vi "CTRE_Phoenix_MotorControl_StartMotionProfile.vi"(7 "BufferedTrajectoryPointStream_DevRef":T2, 8 "error in":errorcluster, 9 "Control Mode":T1=6 items=["MotionProfile"=6, "MotionProfileArc"=10], 10 "minBufferedPts":u32, 11 "PhoenixMotorControlDevRef":T3={"DeviceStatus"={"status"=FALSE, "code"=0, "source"=""}, "Type"=enum."PWM", "PWM"={"PWM Channel"=enum."Invalid", "DeadBand"={"Name"="", "maxPositivePwm"=0, "minPositivePwm"=0, "centerPwm"=0, "maxNegativePwm"=0, "minNegativePwm"=0, "angularRange"=0}}, "CAN"={"Device Number"=0, "SetOutput VI Ref"=variant(enum8{"Percent VBus", "Current", "Speed", "Position", "Voltage"} enum."Percent VBus"), "GetOutput VI Ref"=variant(refnum<k1> refnum), "Enable VI Ref"=variant(dbl 12.0), "Disable VI Ref"=variant(enum8{"Percent VBus", "Speed", "Position", "Slave", "Unchanged / Invalid", "Voltage Compensation", "Current", "Motion Profile"} enum."Percent VBus"), "Data"=variant}, "Invert"=FALSE, "DIO PWM"={"PWM \"Enable\" Channel"=enum."Invalid", "DIOChannel"=enum."Invalid", "PWM Rate"=0.0}}) -> (0 "error out":errorcluster, 3 "PhoenixMotorControlDevRef":T3={"DeviceStatus"={"status"=FALSE, "code"=0, "source"=""}, "Type"=enum."PWM", "PWM"={"PWM Channel"=enum."Invalid", "DeadBand"={"Name"="", "maxPositivePwm"=0, "minPositivePwm"=0, "centerPwm"=0, "maxNegativePwm"=0, "minNegativePwm"=0, "angularRange"=0}}, "CAN"={"Device Number"=0, "SetOutput VI Ref"=variant(enum8{"Percent VBus", "Current", "Speed", "Position", "Voltage"} enum."Percent VBus"), "GetOutput VI Ref"=variant(refnum<k1> refnum), "Enable VI Ref"=variant(dbl 12.0), "Disable VI Ref"=variant(enum8{"Percent VBus", "Speed", "Position", "Slave", "Unchanged / Invalid", "Voltage Compensation", "Current", "Motion Profile"} enum."Percent VBus"), "Data"=variant}, "Invert"=FALSE, "DIO PWM"={"PWM \"Enable\" Channel"=enum."Invalid", "DIOChannel"=enum."Invalid", "PWM Rate"=0.0}})   [LabVIEW 2018]
doc: "Simple one-shot firing of a complete MP.\nStarting in 2019, MPs can be fired by building a Buffered Trajectory Point Stream, and calling this routine.\n\nOnce called, the motor controller software will automatically ...\n[1] Clear the firmware buffer of trajectory points.\n[2] Clear the underrun flags\n[3] Reset an index within the Buffered Trajectory Point Stream (so that the same profile can be run again and again).\n[4] Start a background thread to manage MP streaming (if not already running).\n[5a] If current control mode already matches motionProfControlMode, set MPE Output to \"Hold\".\n[5b] If current control mode does not matches motionProfControlMode, apply motionProfControlMode and set MPE Output to \"Disable\".\n[6] Stream the trajectory points into the device's firmware buffer.\n[7] Once motor controller has at least minBufferedPts worth in the firmware buffer, MP will automatically start (MPE Output set to \"Enable\").\n[8] Wait until MP finishes, then transitions the Motion Profile Executor's output to \"Hold\".\n[9] IsMotionProfileFinished() will now return true.\n\nCalling application can use IsMotionProfileFinished() to determine when internal state machine reaches [7].\nCalling application can cancel MP by calling set(). Otherwise do not call set() until MP has completed.\n\nThe legacy API from previous years requires the calling application to pass points via the ProcessMotionProfileBuffer and PushMotionProfileTrajectory.\nThis is no longer required if using this StartMotionProfile/IsMotionProfileFinished API.\n\n <b>Buffered Trajectory Point Stream</b> A buffer that will be used to stream the trajectory points. Caller can fill this container with the entire trajectory point, regardless of size.\n <b>minBufferedPts</b> Minimum number of firmware buffered points before starting MP. \n Do not exceed device's firmware buffer capacity or MP will never fire (120 for Motion Profile, or 60 for Motion Profile Arc).\n Recommendation value for this would be five to ten samples depending on timeDur of the trajectory point.\n <b>motionProfControlMode</b> Pass MotionProfile or MotionProfileArc."
uses:
  <vilib>/Rock Robotics/WPI/MotorControl/WPI_MotorControlDeviceRef.ctl
  <vilib>/Rock Robotics/WPI/MotorControl/WPI_MotorControlType.ctl
  <vilib>/Rock Robotics/SystemInterfaces/DIO/FPGA_DIOPWMChannel.ctl
  <vilib>/Rock Robotics/WPI/PWM/WPI_PWMDeadband.ctl
  <vilib>/Rock Robotics/SystemInterfaces/DIO/FPGA_DIOChannel.ctl
  <vilib>/Rock Robotics/WPI/ThirdParty/Phoenix-LabVIEW/Motor Controller/Controls/CTRE_Phoenix_MotorControl_BufferedTrajectoryPointStream_DeviceRef.ctl
  <vilib>/Rock Robotics/WPI/ThirdParty/Phoenix-LabVIEW/Motor Controller/Controls/CTRE_Phoenix_MotorControl_MotionProfileControlMode.ctl
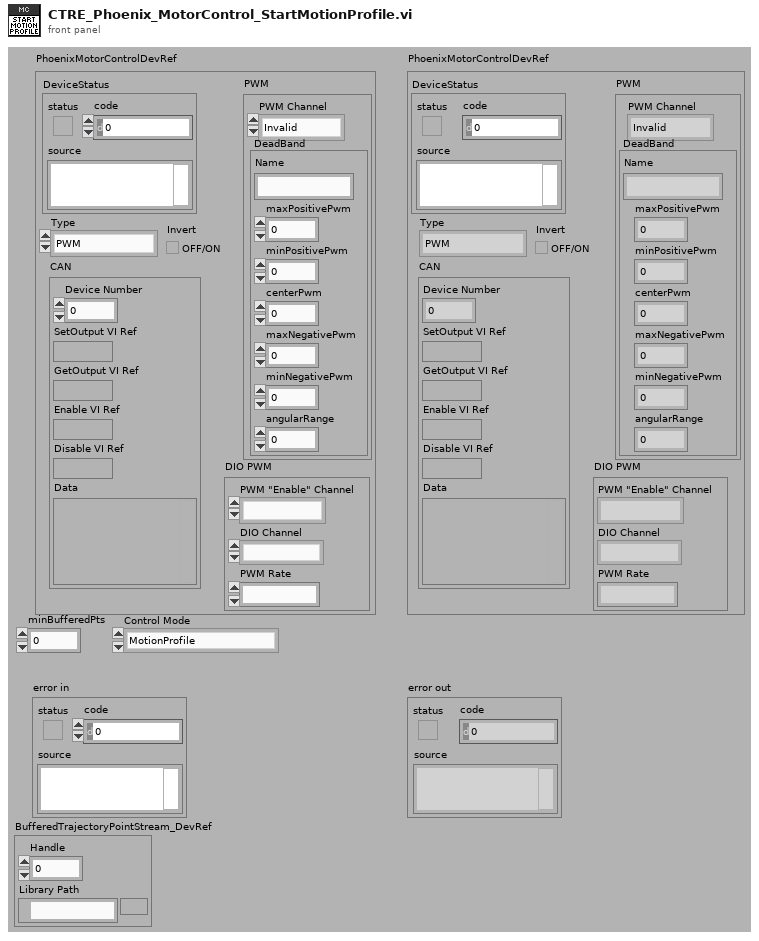
[diagram p1: front panel]
types:
  T1 = typedef "CTRE_Phoenix_MotorControl_MotionProfileControlMode.ctl" = u16
  T2 = typedef "CTRE_Phoenix_MotorControl_BufferedTrajectoryPointStream_DeviceRef.ctl" = cluster{"Handle":u64, "Library Path":path}
  T3 = typedef "WPI_MotorControlDeviceRef.ctl" = cluster{"DeviceStatus":errorcluster, "Type":T4, "PWM":cluster{"PWM Channel":T5, "DeadBand":T6}, "CAN":cluster{"Device Number":u8, "SetOutput VI Ref":variant, "GetOutput VI Ref":variant, "Enable VI Ref":variant, "Disable VI Ref":variant, "Data":variant}, "Invert":bool, "DIO PWM":cluster{"PWM \"Enable\" Channel":T5, "DIOChannel":T7, "PWM Rate":dbl}}
  T4 = typedef "WPI_MotorControlType.ctl" = enum16{"PWM", "CAN", "DIO PWM"}
  T5 = typedef "FPGA_DIOPWMChannel.ctl" = enum8{"PWM 0", "PWM 1", "PWM 2", "PWM 3", "PWM 4", "PWM 5", "PWM 6", "PWM 7", "PWM 8", "PWM 9", "PWM MXP 0", "PWM MXP 1", "PWM MXP 2", "PWM MXP 3", "PWM MXP 4", "PWM MXP 5", "PWM MXP 6", "PWM MXP 7", "PWM MXP 8", "PWM MXP 9", "Invalid"}
  T6 = typedef "WPI_PWMDeadband.ctl" = cluster{"Name":string, "maxPositivePwm":i32, "minPositivePwm":i32, "centerPwm":i32, "maxNegativePwm":i32, "minNegativePwm":i32, "angularRange":u16}
  T7 = typedef "FPGA_DIOChannel.ctl" = enum8{"DIO 0", "DIO 1", "DIO 2", "DIO 3", "DIO 4", "DIO 5", "DIO 6", "DIO 7", "DIO 8", "DIO 9", "DIO MXP 0", "DIO MXP 1", "DIO MXP 2", "DIO MXP 3", "DIO MXP 4", "DIO MXP 5", "DIO MXP 6", "DIO MXP 7", "DIO MXP 8", "DIO MXP 9", "DIO MXP 10", "DIO MXP 11", "DIO MXP 12", "DIO MXP 13", "DIO MXP 14", "DIO MXP 15", "SPI Port CS1", "SPI Port CS2", "SPI Port CS3", "SPI Port MISO", "SPI Port MOSI", "Invalid"}
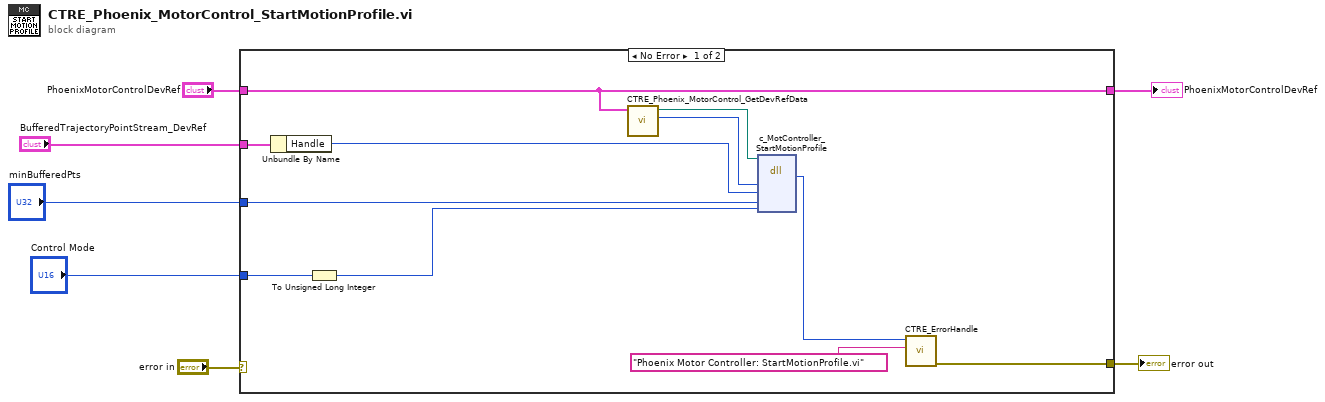
[diagram p0: block diagram]
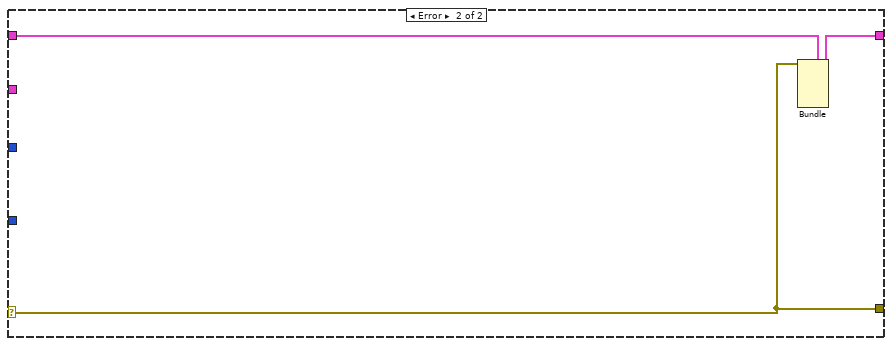
[diagram p2: hidden frame]
diagram:
  n1 = case shown="No Error" "error in" {
    selector: "error in" -> [_ w20]
    tunnel: "PhoenixMotorControlDevRef" -> [w18 w21]
    tunnel: [w15 w20] -> w6
    tunnel: [w18 w19] -> w4
    tunnel: "BufferedTrajectoryPointStream_DevRef" -> [w12 _]
    tunnel: "minBufferedPts" -> [w10 _]
    tunnel: "Control Mode" -> [w9 _]
    frame No Error {
      n2 = Unbundle By Name(w12) -> ("Handle"=w11:u64)
      n3 = To Unsigned Long Integer(number=w9) -> (unsigned 32bit integer=w8:u32)
      n4 = call <vilib>:"CTRE_Phoenix_MotorControl_GetDevRefData.vi"("PhoenixMotorControlDevRef"=w18) -> ("handle"=w16:u64, "Library"=w17:path)  [unwired: 4 in, 5 out]
      n5 = dll-call lib="?" fn="c_MotController_StartMotionProfile"(path in=w17, "handle"=w16, "streamHandle"=w11, "minBufferedPts"=w10, "controlMode"=w8) -> ("ErrorCode"=w14:i32)  [unwired: 6 in, 2 out]
      n6 = call <vilib>:"CTRE_ErrorHandle.vi"("origin"="Phoenix Motor Controller: StartMotionProfile.vi", "code"=w14) -> ("error out"=w15:errorcluster)  [unwired: 9 in]
    }
    frame Error {
      n7 = Bundle(cluster=w21, "DeviceStatus"=w20) -> (w19:T3)  [unwired: 5 in]
    }
  }
  "PhoenixMotorControlDevRef" <- w4
  "error out" <- w6
